vi "程序全局.vi"() -> ()   [LabVIEW 2014]
panel:
  out "小信号变比":cluster{"UB":sgl, "IB":sgl, "UC":sgl, "IA":sgl}
  out "电能表参数数组":T1(array[cluster])=[{"有功常数"=0, "无功常数"=0, "校验圈数"=5, "校验类型"=0, "S值计算次数"=0, "S值计算方法"=0}, {"有功常数"=0, "无功常数"=0, "校验圈数"=5, "校验类型"=0, "S值计算次数"=0, "S值计算方法"=0}, {"有功常数"=0, "无功常数"=0, "校验圈数"=5, "校验类型"=0, "S值计算次数"=0, "S值计算方法"=0}]
  in  "标定电流":sgl
  in  "额定电压":sgl
  in  "有效状态":u8
  out "电能信息":T2
  in  "误差限值":sgl
  in  "电流输出":sgl
  in  "电压输出":sgl
  out "本机表参数":cluster{"有功常数":i32, "无功常数":i32, "输出类型":i32}
  in  "脉冲输入口":u8
  out "电能表参数":T3
  in  "电流档位":u32 format="%.0x"
  in  "电压档位":u32 format="%.0x"
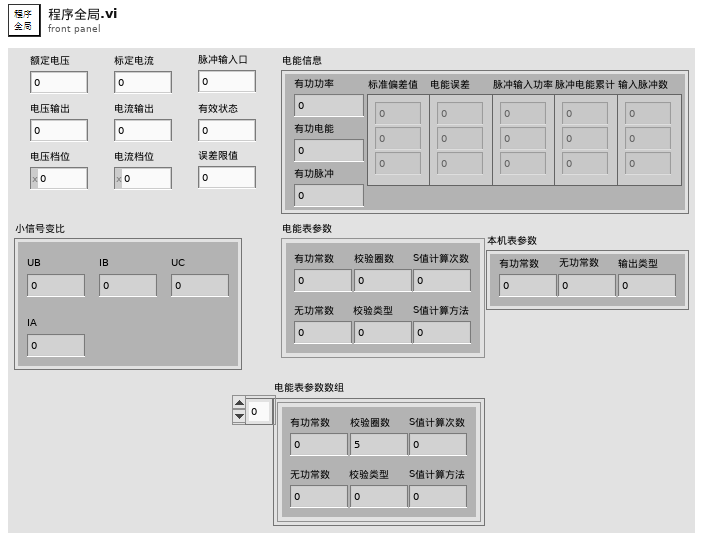
[diagram p1: front panel]
types:
  T1 = cluster{"有功常数":i32, "无功常数":i32, "校验圈数":i32, "校验类型":i32, "S值计算次数":i32, "S值计算方法":i32}[]
  T2 = cluster{"有功功率":sgl, "有功电能":sgl, "有功脉冲":u64, "标准偏差值":sgl[], "电能误差":sgl[], "脉冲输入功率":sgl[], "脉冲电能累计":sgl[], "输入脉冲数":sgl[]}
  T3 = cluster{"有功常数":i32, "无功常数":i32, "校验圈数":i32, "校验类型":i32, "S值计算次数":i32, "S值计算方法":i32}
diagram:
